vi "DCMotor_GetSpeed.vi"(9 "VoltageInput_Volts":dbl format="%13.5p", 10 "torque_Nm":dbl format="%13.5p", 11 "DCMOTOR":T1 {"Jr_KgM2" format="%13.5p"; "L_H" format="%13.5p"; "Kt_NMPerAmp" format="%13.5p"; "KvINV_RadPerSecPerVolt" format="%13.5p"; "R_Ohms" format="%13.5p"; "FreeSpeed_RadPerSec" format="%13.5p"; "FreeCurrent_Amps" format="%13.5p"; "StallCurrent_Amps" format="%13.5p"; "StallTorque_NM" format="%13.5p"; "nominalVoltage_Volts" format="%13.5p"}) -> (3 "Speed_Rad/Sec":dbl format="%13.5p")   [LabVIEW 2019, in "Trajectory_Library.lvlib"]
doc: "Calculate the speed of the mtor given torque and voltage input.\n\nInputs: \n - DCMOTOR -- Cluster containing the motor modeling constants for this set of motors.\n - Torque -- The torque produced by the motor. (NM)\n - Voltage -- The voltage applied to the motor. (Volts)\n\nOutputs:\n - Speed -- double -- Motor speed (Rad/Sec)"
uses:
  TypeDef/DCMOTOR.CTL
  Trajectory_Library.lvlib
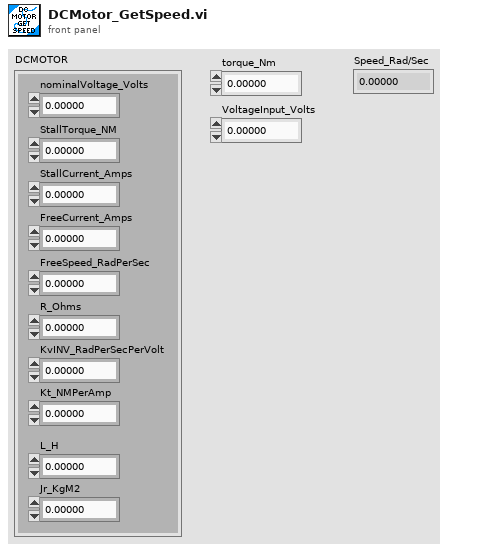
[diagram p1: front panel]
types:
  T1 = typedef "Trajectory_Library.lvlib/DCMOTOR.CTL" = cluster{"nominalVoltage_Volts":dbl, "StallTorque_NM":dbl, "StallCurrent_Amps":dbl, "FreeCurrent_Amps":dbl, "FreeSpeed_RadPerSec":dbl, "R_Ohms":dbl, "KvINV_RadPerSecPerVolt":dbl, "Kt_NMPerAmp":dbl, "L_H":dbl, "Jr_KgM2":dbl}
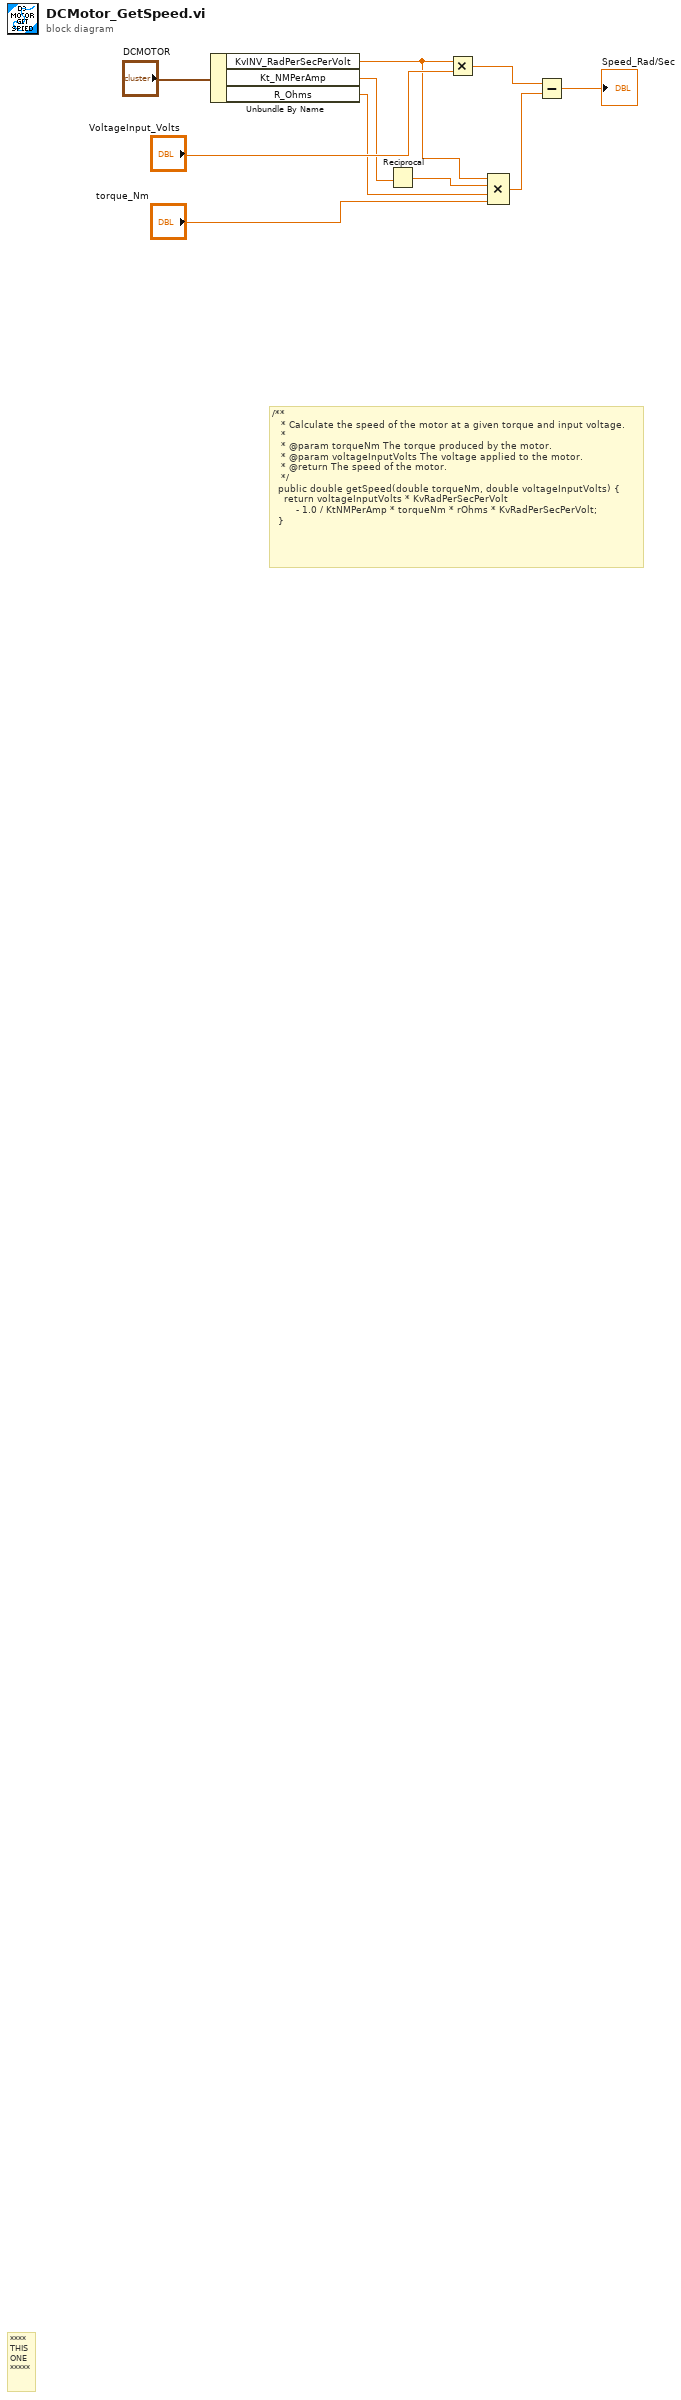
[diagram p0: block diagram]
diagram:
  # "/**\n   * Calculate the speed of the motor at a given torque and input voltage.\n   *\n   * @param torqueNm The torque produced by the motor.\n   * @param voltageInputVolts The voltage applied to the motor.\n   * @return The speed of the motor.\n   */\n  public double getSpeed(double torqueNm, double voltageInputVolts) {\n    return voltageInputVolts * KvRadPerSecPerVolt\n        - 1.0 / KtNMPerAmp * torqueNm * rOhms * KvRadPerSecPerVolt;\n  }"
  # "****\nTHIS\nONE\n*****"
  n1 = Unbundle By Name("DCMOTOR") -> ("KvINV_RadPerSecPerVolt"=w7:dbl, "Kt_NMPerAmp"=w6:dbl, "R_Ohms"=w4:dbl)
  n2 = Reciprocal(x=w6) -> (1/x=w5:dbl)
  n3 = Multiply(x=w7, y="VoltageInput_Volts") -> (x*y=w8:dbl)
  n4 = Compound Arithmetic op=MULTIPLY(w7, w5, w4, "torque_Nm") -> (w2:dbl)
  n5 = Subtract(x=w8, y=w2) -> (x-y=→"Speed_Rad/Sec":dbl)
